vi "SimpleAdd.vi"() -> ()   [LabVIEW 2018]
panel:
  out "x+y":dbl
  in  "x":dbl
  in  "y":dbl
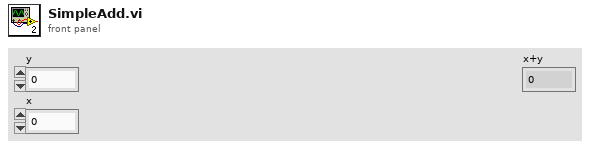
[diagram p1: front panel]
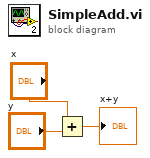
[diagram p0: block diagram]
diagram:
  n1 = Add(x="x", y="y") -> (x+y=→"x+y":dbl)
